vi "Throw Error - Impossible Initial State - Reason 3.vi"(8 "error in":errorcluster) -> (0 "error out":errorcluster)   [LabVIEW 2022 SP3]
doc: "Throws a user-generated error that indicates that an impossible initial state was detected."
panel:
  # "Development\ncontrols/indicators useful for development and testing, but which are not outputs of the VI"
  # "Input\nInputs to the VI"
  # "Output\nOutputs of the VI"
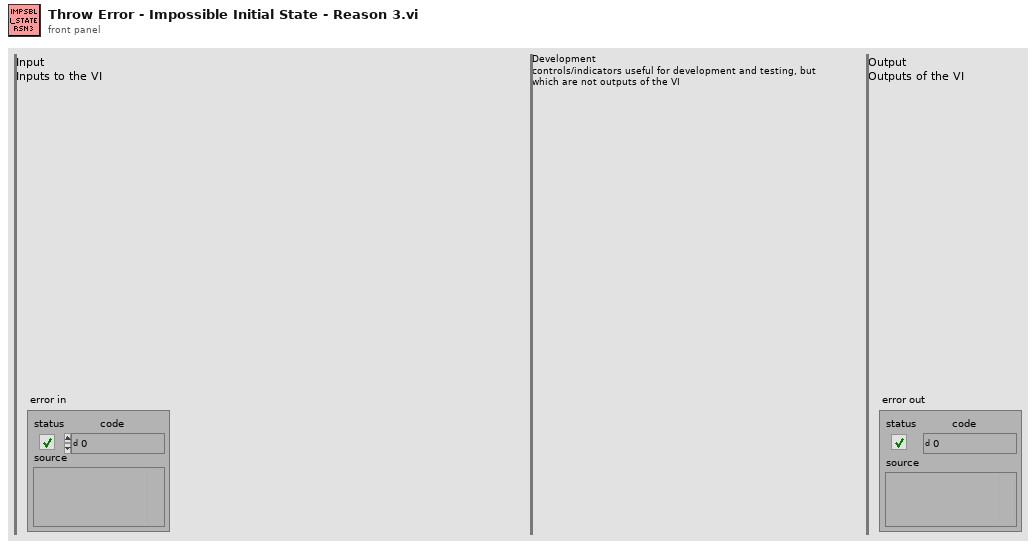
[diagram p1: front panel]
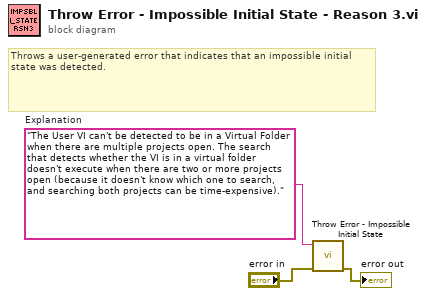
[diagram p0: block diagram]
diagram:
  w3 = "The User VI can't be detected to be in a Virtual Folder when there are multiple projects open. The search that detects whether the VI is in a virtual folder doesn't execute when there are two or more projects open (because it doesn't know which one to search, and searching both projects can be time-expensive)."  # Explanation
  # "Throws a user-generated error that indicates that an impossible initial state was detected."
  n1 = call "Throw Error - Impossible Initial State.vi"("error in"="error in", "Explanation"=w3) -> ("error out"=→"error out":errorcluster)  [unwired: 9 in]
